vi "initialize(picture).vi"(11 "picture size":dbl) -> (3 "2D Picture":picture)   [LabVIEW 2022 SP3, in "drawPlate.lvlib"]
uses:
  drawPlate.lvlib
panel:
  # "根據圖片大小畫下一開始的棋盤(中央有黑白各二子交錯)"
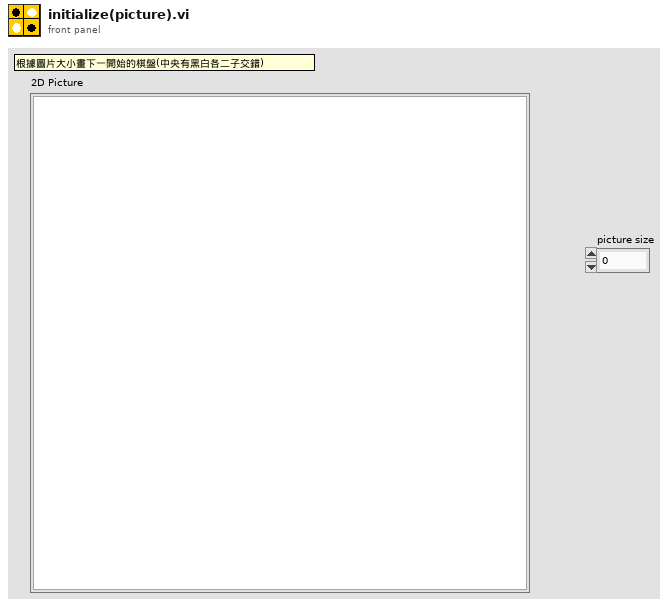
[diagram p1: front panel]
types:
  T1 = cluster{i32, i32, "picture size":dbl, "picture size":dbl}
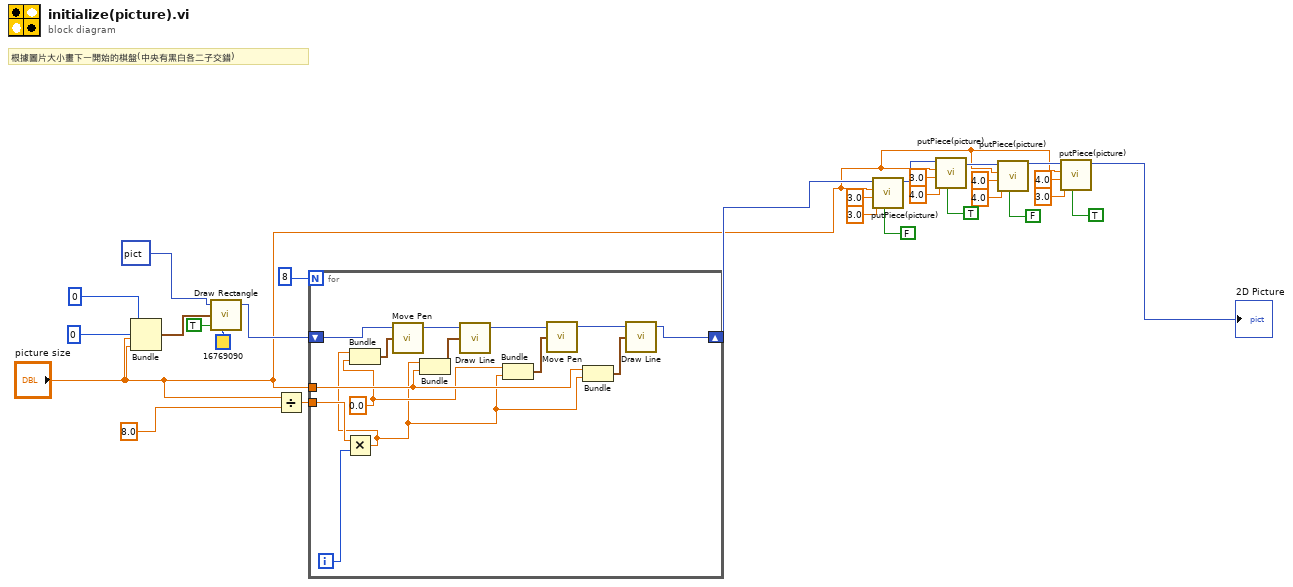
[diagram p0: block diagram]
diagram:
  # "根據圖片大小畫下一開始的棋盤(中央有黑白各二子交錯)"
  n1 = Bundle(0, 0, "picture size"="picture size", "picture size"="picture size") -> (w19:T1)  [unwired: 1 in]
  n2 = call <vilib>:"Draw Rectangle.vi"("picture"=picture data[5B] ("2D Picture"), "rect"=w19, "fill?(F)"=TRUE, "color(black)"=u32 16769090) -> ("new picture"=w24:picture)  [unwired: 5 in]
  n3 = Divide(x="picture size", y=8.0) -> (x/y=w27:dbl)
  n4 = for {
    N: 8 -> [_]
    tunnel: w27 -> [w42]
    shift-right: [w36] -> w2
    shift-left: w24 -> [w40]
    tunnel: "picture size" -> [w31]
    i -> [w41]
    w30 = 0.0
    n5 = Multiply(x=w42, y=w41) -> (x*y=w29:dbl)
    n6 = Bundle(w29, w30) -> (w32:cluster{dbl, dbl})  [unwired: 1 in]
    n7 = call <vilib>:"Move Pen.vi"("new position"=w32, "picture"=w40) -> ("new picture"=w39:picture)  [unwired: 3 in]
    n8 = Bundle(w29, "picture size"=w31) -> (w33:cluster{dbl, "picture size":dbl})  [unwired: 1 in]
    n9 = call <vilib>:"Draw Line.vi"("picture"=w39, "end point"=w33) -> ("new picture"=w38:picture)  [unwired: 7 in]
    n10 = Bundle(w30, w29) -> (w34:cluster{dbl, dbl})  [unwired: 1 in]
    n11 = call <vilib>:"Move Pen.vi"("new position"=w34, "picture"=w38) -> ("new picture"=w37:picture)  [unwired: 3 in]
    n12 = Bundle("picture size"=w31, w29) -> (w35:cluster{"picture size":dbl, dbl})  [unwired: 1 in]
    n13 = call <vilib>:"Draw Line.vi"("picture"=w37, "end point"=w35) -> ("new picture"=w36:picture)  [unwired: 7 in]
  }
  n14 = call "putPiece(picture).vi"("drawRed"=FALSE ("is black's turn?"), "posy"=3.0, "posx"=3.0, "picture size"="picture size", "2D Picture 2"=w2) -> ("2D Picture"=w18:picture)  [unwired: 6 in]
  n15 = call "putPiece(picture).vi"("drawRed"=TRUE ("is black's turn?"), "posy"=4.0, "posx"=3.0, "picture size"="picture size", "2D Picture 2"=w18) -> ("2D Picture"=w17:picture)  [unwired: 6 in]
  n16 = call "putPiece(picture).vi"("drawRed"=FALSE ("is black's turn?"), "posy"=4.0, "posx"=4.0, "picture size"="picture size", "2D Picture 2"=w17) -> ("2D Picture"=w16:picture)  [unwired: 6 in]
  n17 = call "putPiece(picture).vi"("drawRed"=TRUE ("is black's turn?"), "posy"=3.0, "posx"=4.0, "picture size"="picture size", "2D Picture 2"=w16) -> ("2D Picture"=→"2D Picture":picture)  [unwired: 6 in]
